vi "Stage Test Launcher.vi"(9 "Sub Panel":refnum<vi>, 11 "Panel Actor In":refnum<class "Main.lvclass">) -> (2 "Nested Actor's Enqueuer":refnum<class "Message Enqueuer.lvclass">, 3 "Panel Actor Out":refnum<class "Main.lvclass">)   [LabVIEW 2018]
uses:
  <vilib>/MGI/Panel Manager/Panel/Panel.lvlib
  <vilib>/MGI/Panel Manager/Panel Actor/Panel Actor/Panel Actor.lvclass
  Stage.lvclass
  <instrlib>/Zaber A Series/Zaber A Series.lvlib
  <vilib>/MGI/Panel Manager/Panel/Panel/Subpanel/Subpanel.vi
  <vilib>/MGI/Panel Manager/Panel/Panel/Subpanel/Subpanel.lvclass
  C:/Program Files/National Instruments/LabVIEW 2018/vi.lib/MGI/Panel Manager/Panel Actor/Panel Actor/Panel Actor.lvclass
  C:/Program Files/National Instruments/LabVIEW 2018/vi.lib/MGI/Monitored Actor/Monitored Actor/Monitored Actor/Monitored Actor.lvclass
  C:/Program Files/National Instruments/LabVIEW 2018/vi.lib/ActorFramework/Actor/Actor.lvclass
  C:/Program Files/National Instruments/LabVIEW 2018/vi.lib/MGI/Panel Manager/Panel/Panel/Panel.lvclass
  ADM/ADM/Main.lvclass
  <vilib>/ActorFramework/Message Enqueuer/Message Enqueuer.lvclass
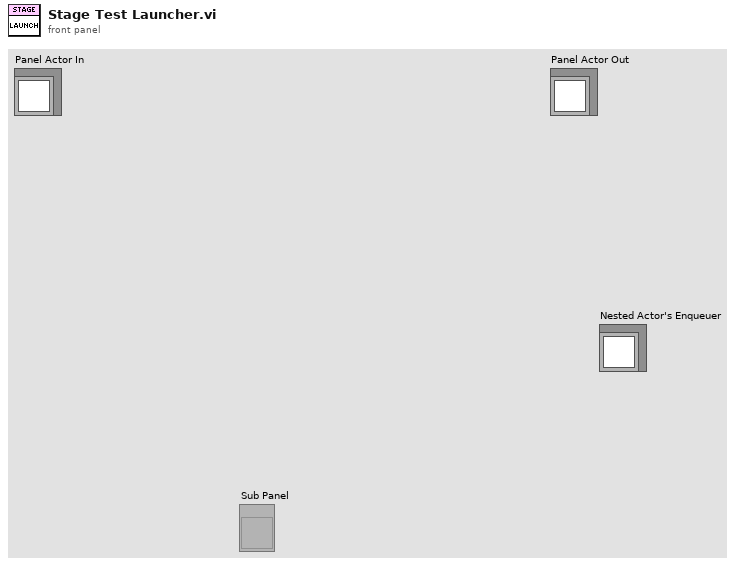
[diagram p1: front panel]
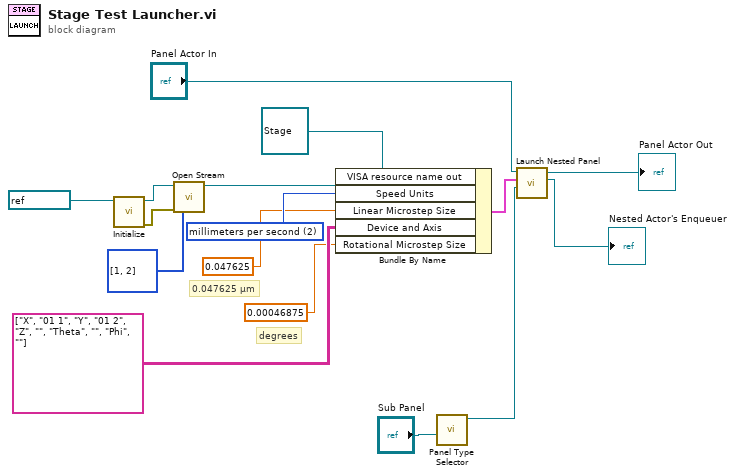
[diagram p0: block diagram]
diagram:
  w5 = u16 2 items=["device speed units", "microns per second", "millimeters per second", "inches per second", "degrees per second"] ("Speed Units")
  # "degrees"
  # "0.047625 µm"
  n1 = call <instrlib>:"Initialize.vi"("VISA resource name"=refnum<visa-resource-name> "COM8") -> ("error out"=w3:errorcluster, "VISA resource name out"=w8:refnum<visa-resource-name>)  [unwired: 9 in]
  n2 = call <instrlib>:"Open Stream.vi"("Axis Numbers (1,2)"=u8[] [1, 2], "error in (no error)"=w3, "VISA resource name"=w8) -> ("VISA resource name out"=w7:refnum<visa-resource-name>)  [unwired: 7 in, 1 out]
  n3 = Bundle By Name(cluster=refnum<class "Stage.lvclass"> refnum ("Stage Actor.lvlib:Stage.lvclass"), "VISA resource name out"=w7, "Speed Units"=w5, "Linear Microstep Size"=0.047625, "Device and Axis"=string[][] [["X", "01 1"], ["Y", "01 2"], ["Z", ""], ["Theta", ""], ["Phi", ""]], "Rotational Microstep Size"=0.00046875) -> (w13:cluster{})
  n4 = call-poly <vilib>:"Panel Type Selector.vi"("Sub Panel"="Sub Panel") -> ("Subpanel Out"=w14:refnum<class "Subpanel.lvclass">)  [unwired: 9 in, 1 out]
  n5 = call <vilib>:"Launch Nested Panel.vi"("Panel"=w14, "Nested Panel Actor"=w13, "Panel Actor in"="Panel Actor In") -> ("Nested Actor's Enqueuer"=→"Nested Actor's Enqueuer":refnum<class "Message Enqueuer.lvclass">, "Panel Actor out"=→"Panel Actor Out":refnum<class "Main.lvclass">)  [unwired: 5 in, 2 out]
